vi "Post-Build Action.vi"(5 "Files Generated by Build":path[](array[path]), 6 "Top Level/Always Included VIs":path[](array[path]), 7 "Destination Path":path, 8 "error in (no error)":errorcluster, 9 "Target Name":string, 10 "Build Specification Name":string, 11 "Project Path":path) -> (0 "error out":errorcluster)   [LabVIEW 2024]
uses:
  <vilib>/Utility/error.llb/Error Cluster From Error Code.vi
  <vilib>/ErrorRing/Error Ring.xnode
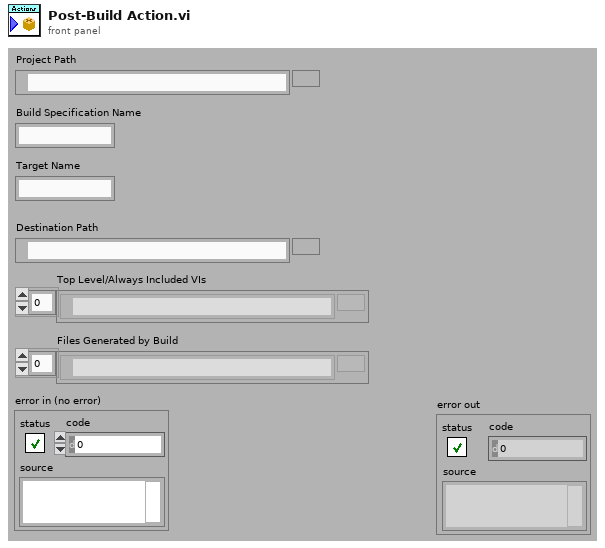
[diagram p1: front panel]
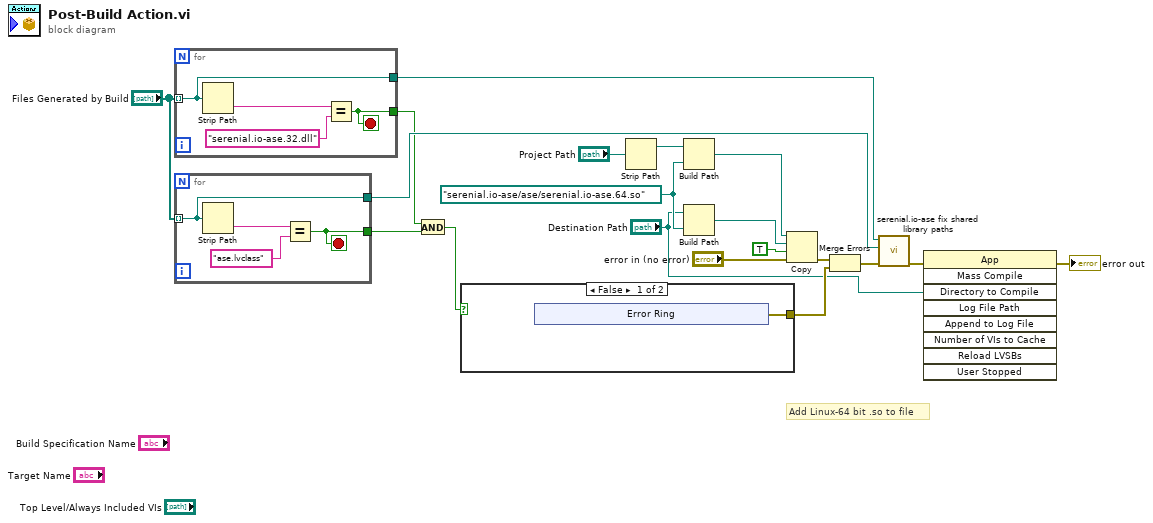
[diagram p0: block diagram]
diagram:
  w17 = path "serenial.io-ase/ase/serenial.io-ase.64.so" ("name or relative path")
  # "Add Linux-64 bit .so to file"
  n1 = for {
    tunnel: "Files Generated by Build" -> [w21] mode=indexing
    tunnel: [w21] -> w10
    tunnel: [w20] -> w9
    stop <- w20 stop-if-true
    n2 = Strip Path(path=w21) -> (name=w23:string)  [unwired: 1 out]
    n3 = Equal?(x=w23, y="serenial.io-ase.32.dll") -> (x = y?=w20:bool)
  }
  n4 = for {
    tunnel: "Files Generated by Build" -> [w25] mode=indexing
    tunnel: [w25] -> w11
    tunnel: [w24] -> w8
    stop <- w24 stop-if-true
    n5 = Strip Path(path=w25) -> (name=w27:string)  [unwired: 1 out]
    n6 = Equal?(x=w27, y="ase.lvclass") -> (x = y?=w24:bool)
  }
  n7 = And(x=w9, y=w8) -> (x .and. y?=w7:bool)
  n8 = case shown="False" w7 {
    tunnel: [w28 _] -> w6
    frame False {
      n9 = xnode "Error Ring"() -> ("error out"=w28:errorcluster)
    }
    frame True {
    }
  }
  n10 = Strip Path(path="Project Path") -> (stripped path=w18:path)  [unwired: 1 out]
  n11 = Build Path(base path=w18, name or relative path=w17) -> (appended path=w16:path)
  n12 = Build Path(base path="Destination Path", name or relative path=w17) -> (appended path=w15:path)
  n13 = Copy(8:"error in (no error)", 9:TRUE ("overwrite (F)"), 10:w15, 11:w16) -> (0:w4:errorcluster)  [unwired: 1 in, 2 out]
  n14 = Merge Errors(w4, w6) -> (w5:errorcluster)
  n15 = call "serenial.io-ase fix shared library paths.vi"("error in"=w5, "class path"=w11, "Shared Library Path"=w10) -> ("error out"=w3:errorcluster)  [unwired: 8 in]
  n16 = invoke class="App" method="Mass Compile"(error in=w3, "Directory to Compile"="Destination Path") -> (error out=→"error out":errorcluster)  [unwired: 7 in, 8 out]
